vi "XY Graph Show-Hide Cursor Axes.vi"(6 "Show Cursor Axes":bool, 8 "Error In":errorcluster, 11 "XYGraph in":refnum<vi>) -> (0 "Error Out":errorcluster)   [LabVIEW 2021, in "XY Graph Add-Ons.lvlib"]
uses:
  XY Graph Add-Ons.lvlib
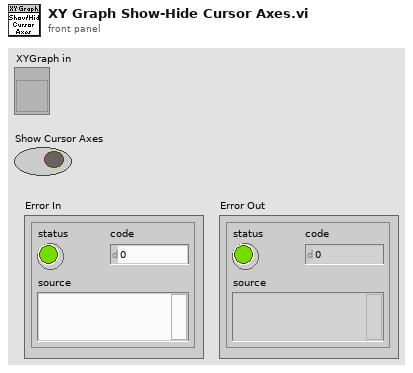
[diagram p1: front panel]
types:
  T1 = typedef "LVCursorListTypeDef.ctl" = cluster{"Name":string, "Color":u32, "Style":u8, "Point Style":u8, "Name Visible":bool, "Allow Drag":bool, "Cursor Mode":u32, "Plot":i32, "Index":i32, "Position":cluster{"X":dbl, "Y":dbl}, "X Scale":u32, "Y Scale":u32, "Watch Plots":i32[], "Watch All Plots":bool, "Plot Area":i32, "Label Offset":cluster{"X":dbl, "Y":dbl}}[]
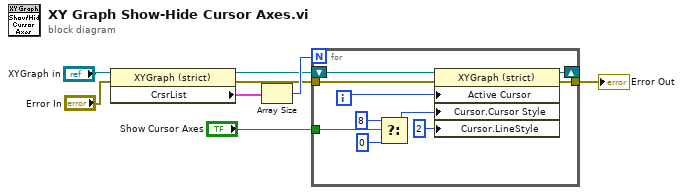
[diagram p0: block diagram]
diagram:
  n1 = property on="Property Node" class="XYGraph (strict)"(reference="XYGraph in", error in="Error In") -> (reference out=w4:refnum<vi>, error out=w2:errorcluster, "CrsrList"=w6:T1)
  n2 = Array Size(array=w6) -> (size(s)=w5:i32)
  n3 = for {
    N: w5 -> [_]
    tunnel: "Show Cursor Axes" -> [w18]
    shift-right: [w14] -> _
    shift-left: w4 -> [w15]
    tunnel: w2 -> [w10]
    tunnel: [w9] -> w1
    i -> [w13]
    n4 = Select(t=u8 8, s=w18, f=u8 0 ("Style")) -> (s? t:f=w12:u8)
    n5 = property on="Property Node" class="XYGraph (strict)"(reference=w15, error in=w10, "Active Cursor"=w13, "Cursor.Cursor Style"=w12, "Cursor.LineStyle"=u8 2 ("Cursor.Line Style")) -> (reference out=w14:refnum<vi>, error out=w9:errorcluster)
  }
  "Error Out" <- w1
